vi "Simple Example.vi"() -> ()   [LabVIEW 2020]
uses:
  CommandTypeDef.ctl
panel:
  out "Value":string
  out "error out":errorcluster
  out "data out":string
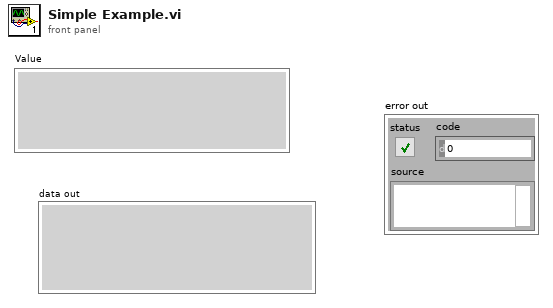
[diagram p1: front panel]
types:
  T1 = typedef "CommandTypeDef.ctl" = enum16{"Current", "MaxVoltage", "SlewRate", "EnableOutput", "Reset", "CurrentVoltage", "MaxCurrent"}
  T2 = enum16{"Standard", "Buffered", "CRLF", "Immediate"}
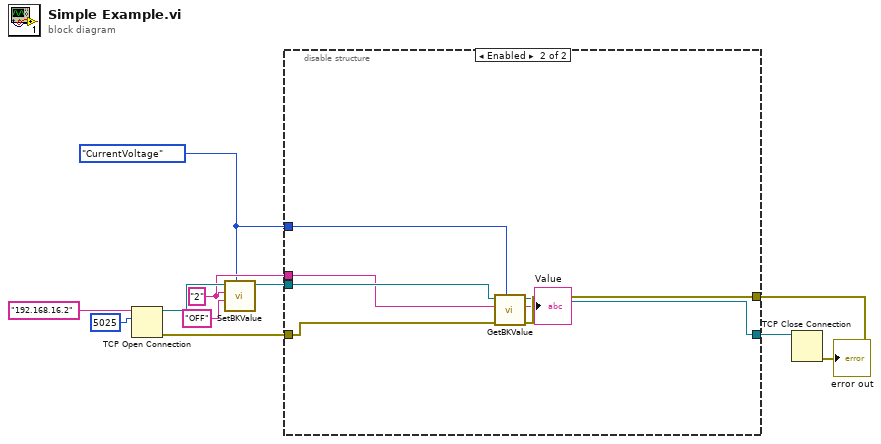
[diagram p0: block diagram]
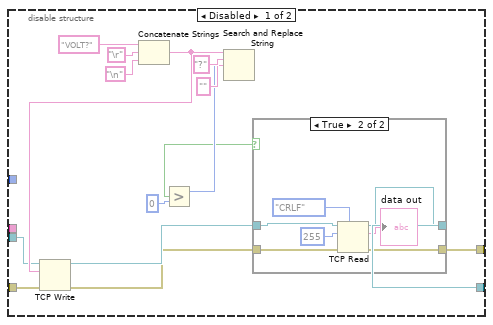
[diagram p2: hidden frame]
diagram:
  w1 = CommandTypeDef."CurrentVoltage" ("Command")
  w2 = "2" ("Channel")
  n1 = TCP Open Connection(address="192.168.16.2", remote port or service name=u16 5025) -> (connection ID=w5:refnum<k5>, error out=w9:errorcluster)  [unwired: 3 in]
  n2 = call "SetBKValue.vi"("Command"=w1, "Value"="OFF", "Channel"=w2, "Connection In"=w5) -> ("Connection Out"=w4:refnum<k5>)  [unwired: 6 in, 1 out]
  n3 = disable-structure shown="Enabled" {
    disable-tunnel: w9 -> [w26 w41]
    disable-tunnel: [w25 w40] -> w8
    disable-tunnel: [w23 w39] -> w7
    disable-tunnel: w4 -> [w12 w42]
    disable-tunnel: w1 -> [_ w38]
    disable-tunnel: w2 -> [_ w37]
    frame Disabled {
      n4 = Concatenate Strings("VOLT?" ("data in"), "\r", "\n") -> (w18:string)
      n5 = TCP Write(connection ID=w12, data in=w18, error in (no error)=w26) -> (connection ID out=w24:refnum<k5>, error out=w19:errorcluster)  [unwired: 1 in, 1 out]
      n6 = Search and Replace String(input string=w18, search string="?", replace string="" ("replace string (\"\")")) -> (number of replacements=w15:i32)  [unwired: 5 in, 3 out]
      n7 = Greater?(x=w15, y=0) -> (0:w13:bool)
      n8 = case shown="True" w13 {
        tunnel: [w27 w35] -> w25
        tunnel: w24 -> [w28 w34]
        tunnel: [w28 w33] -> w23
        tunnel: w19 -> [w27 w29]
        frame False {
        }
        frame True {
          n9 = TCP Read(connection ID=w34, bytes to read=255, error in (no error)=w29, 7:T2."CRLF" ("mode (standard)")) -> (connection ID out=w33:refnum<k5>, data out=→"data out":string, error out=w35:errorcluster)  [unwired: 1 in]
        }
      }
    }
    frame Enabled {
      n10 = call "GetBKValue.vi"("Command"=w38, "error in (no error)"=w41, "Channel"=w37, "Connection In"=w42) -> ("error out"=w40:errorcluster, "Value"=→"Value":string, "Connection Out"=w39:refnum<k5>)  [unwired: 5 in]
    }
  }
  n11 = TCP Close Connection(connection ID=w7, error in (no error)=w8) -> (error out=→"error out":errorcluster)  [unwired: 1 in, 1 out]
